vi "Create Test for All Methods.vi"(8 "error in (no error)":errorcluster, 9 "TestCase Class Path":path=path "C:/Documents and Settings/Administrator/Desktop/Plugin Development/VI Tester Plugin/MyTestCase/testExample.vit", 10 "Class Path":path=path "C:/Documents and Settings/Administrator/Desktop/Plugin Development/VI Tester Plugin/MyTestCase/testExample.vit", 11 "App reference":refnum<vi>) -> (0 "error out":errorcluster, 2 "Invalid methods":path[](array[path]))   [LabVIEW 2010]
uses:
  <userlib>/_OpenG.lib/array/array.llb/Conditional Auto-Indexing Tunnel (Path)__ogtk.vi
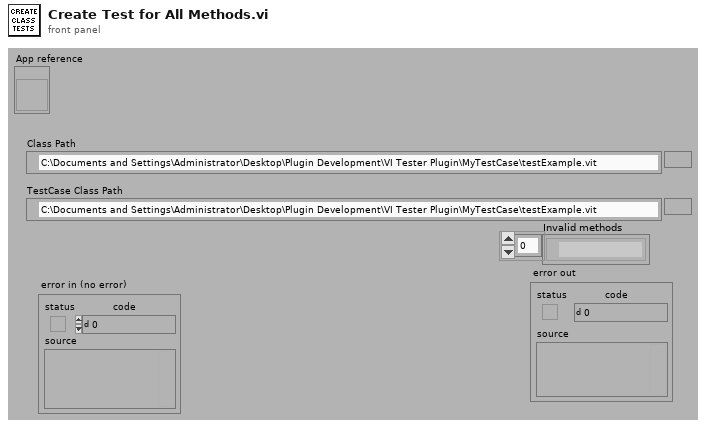
[diagram p1: front panel]
types:
  T1 = enum32{"invalid scope", "public", "private", "protected", "community"}
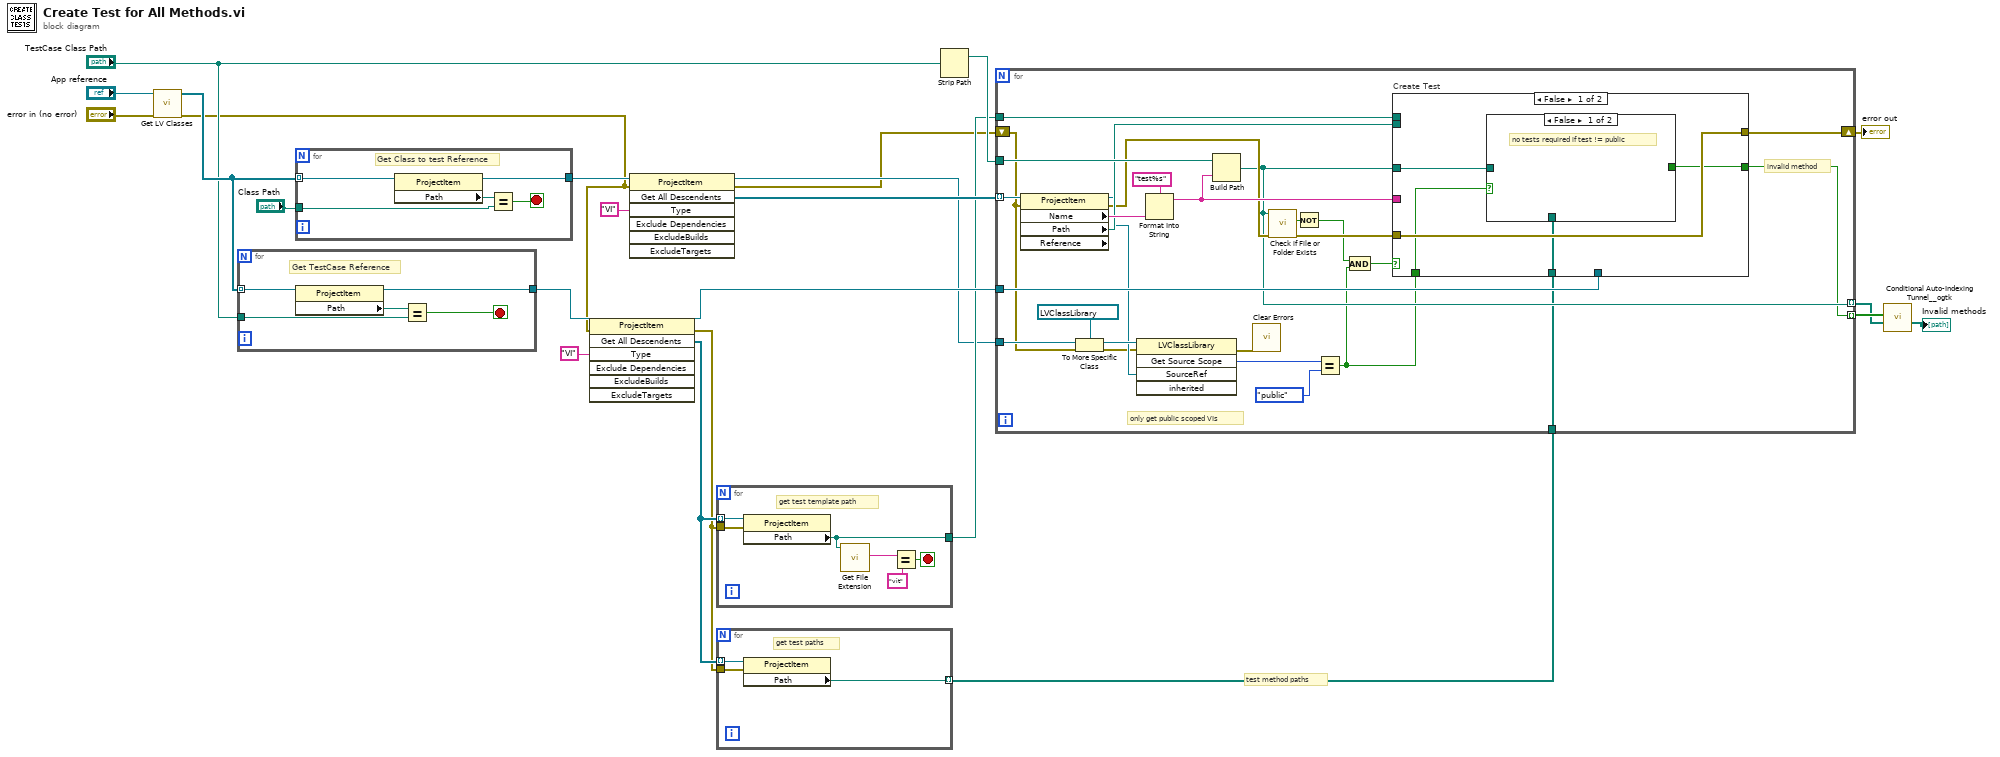
[diagram p0: block diagram]
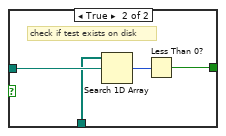
[diagram p2: hidden frame]
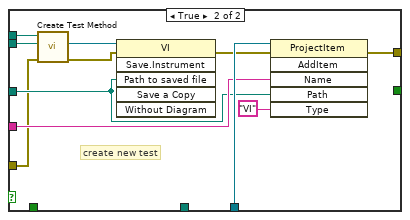
[diagram p3: hidden frame]
diagram:
  # "test method paths"
  n1 = call "Get LV Classes.vi"("error in (no error)"="error in (no error)", "App reference"="App reference") -> ("error out"=w10:errorcluster, "LabVIEW Classes"=w19:refnum<vi>[])  [unwired: 8 in]
  n2 = for {
    tunnel: w19 -> [w28] mode=indexing
    tunnel: "TestCase Class Path" -> [w26]
    tunnel: [w24] -> w13
    stop <- w25 stop-if-true
    # "Get TestCase Reference"
    n3 = property class="ProjectItem"(reference=w28) -> (reference out=w24:refnum<vi>, "Path"=w27:path)  [unwired: 1 in, 1 out]
    n4 = Equal?(x=w27, y=w26) -> (x = y?=w25:bool)
  }
  n5 = for {
    tunnel: w19 -> [w33] mode=indexing
    tunnel: "Class Path" -> [w31]
    tunnel: [w29] -> w22
    stop <- w30 stop-if-true
    # "Get Class to test Reference"
    n6 = property class="ProjectItem"(reference=w33) -> (reference out=w29:refnum<vi>, "Path"=w32:path)  [unwired: 1 in, 1 out]
    n7 = Equal?(x=w32, y=w31) -> (x = y?=w30:bool)
  }
  n8 = invoke class="ProjectItem" method="Get All Descendents"(reference=w13, error in=w10, "Type"="VI") -> (reference out=w12:refnum<vi>, error out=w3:errorcluster, "All Descendents"=w4:refnum<vi>[])  [unwired: 4 in, 4 out]
  n9 = invoke class="ProjectItem" method="Get All Descendents"(reference=w22, error in=w10, "Type"="VI") -> (reference out=w8:refnum<vi>, error out=w1:errorcluster, "All Descendents"=w20:refnum<vi>[])  [unwired: 4 in, 4 out]
  n10 = for {
    tunnel: w4 -> [w39] mode=indexing
    tunnel: [w35] -> w11
    tunnel: w3 -> [w34]
    stop <- w36 stop-if-true
    # "get test template path"
    n11 = property class="ProjectItem"(reference=w39, error in=w34) -> ("Path"=w35:path)  [unwired: 2 out]
    n12 = call <vilib>:"Get File Extension.vi"("file"=w35) -> ("lowercase file extension"=w38:string)  [unwired: 7 in, 3 out]
    n13 = Equal?(x=w38, y="vit") -> (x = y?=w36:bool)
  }
  n14 = for {
    tunnel: w4 -> [w42] mode=indexing
    tunnel: [w41] -> w2 mode=indexing
    tunnel: w3 -> [w40]
    # "get test paths"
    n15 = property class="ProjectItem"(reference=w42, error in=w40) -> ("Path"=w41:path)  [unwired: 2 out]
  }
  n16 = Strip Path(path="TestCase Class Path") -> (stripped path=w17:path)  [unwired: 1 out]
  n17 = for {
    tunnel: w20 -> [w67] mode=indexing
    tunnel: w11 -> [w69]
    tunnel: w12 -> [w68]
    tunnel: w17 -> [w64]
    shift-right: [w62] -> w16
    shift-left: w1 -> [w52]
    tunnel: w8 -> [w56]
    tunnel: [w44] -> w7 mode=indexing
    tunnel: [w47] -> w6 mode=indexing
    tunnel: w2 -> [w45]
    # "invalid method"
    # "only get public scoped VIs"
    n18 = property class="ProjectItem" props=["Name", "Path", "Reference"](reference=w67, error in=w52) -> (reference out=w55:refnum<vi>, error out=w60:errorcluster, "Name"=w65:string, "Path"=w61:path)  [unwired: 1 out]
    n19 = To More Specific Class(target class=refnum<vi> refnum ("reference out"), reference=w56, error in=w52) -> (specific class reference=w57:refnum<vi>, error out=w51:errorcluster)
    n20 = invoke class="LVClassLibrary" method="Get Source Scope"(reference=w57, error in=w51, "SourceRef"=w55) -> (error out=w50:errorcluster, "GetSourceScope"=w46:T1)  [unwired: 2 in, 3 out]
    n21 = Format Into String(format string="test%s", w65) -> (resulting string=w63:string)  [unwired: 2 in, 1 out]
    n22 = Build Path(base path=w64, name or relative path=w63) -> (appended path=w47:path)
    n23 = call <vilib>:"Clear Errors.vi"("error in (no error)"=w50) -> ()  [unwired: 6 in, 1 out]
    n24 = call <vilib>:"Check if File or Folder Exists.vi"("error in (no error)"=w60, "path"=w47) -> ("error out"=w59:errorcluster, "file or folder exists?"=w48:bool)  [unwired: 7 in, 1 out]
    n25 = Not(x=w48) -> (.not. x?=w49:bool)
    n26 = Equal?(x=w46, y=T1."public") -> (x = y?=w43:bool)
    n27 = And(x=w49, y=w43) -> (x .and. y?=w53:bool)
    n28 = case "Create Test" shown="False" w53 {
      tunnel: w69 -> [_ w89]
      tunnel: w68 -> [_ w87]
      tunnel: w63 -> [_ w84]
      tunnel: [w74 w83] -> w62
      tunnel: w61 -> [_ w82]
      tunnel: w47 -> [w73 w80]
      tunnel: w59 -> [w74 w79]
      tunnel: w45 -> [w72 _]
      tunnel: [w71 _] -> w44
      tunnel: w43 -> [w70 _]
      frame False {
        n29 = case shown="False" w70 {
          tunnel: w73 -> [_ w78]
          tunnel: w72 -> [_ w77]
          tunnel: [_ w75] -> w71
          frame False {
            # "no tests required if test != public"
          }
          frame True {
            # "check if test exists on disk"
            n30 = Search 1D Array(1D array=w77, element=w78) -> (index of element=w76:i32)  [unwired: 1 in]
            n31 = Less Than 0?(x=w76) -> (x < 0?=w75:bool)
          }
        }
      }
      frame True {
        # "create new test"
        n32 = call "Create Test Method.vi"("error in"=w79, "Replacement VI"=w82, "template test VI"=w89) -> ("error out"=w81:errorcluster, "New VI Refnum"=w86:refnum<vi>)  [unwired: 7 in]
        n33 = invoke class="VI" method="Save.Instrument"(reference=w86, error in=w81, "Path to saved file"=w80) -> (error out=w85:errorcluster)  [unwired: 3 in, 5 out]
        n34 = invoke class="ProjectItem" method="AddItem"(reference=w87, error in=w85, "Name"=w84, "Path"=w80, "Type"="VI") -> (error out=w83:errorcluster)  [unwired: 1 in, 5 out]
      }
    }
  }
  "error out" <- w16
  n35 = call-poly <userlib>:"Conditional Auto-Indexing Tunnel__ogtk.vi"("Array in"=w6, "Elements to keep"=w7) -> ("Filtered Array out"=→"Invalid methods":path[])  [unwired: 5 in]
